vi "load_standards.vi"(10 "Standards Tree ref":refnum<vi>) -> ()   [LabVIEW 2017]
doc: "loads the Standards information from the StabdardsObjects (NOT from the Standards.ini)"
uses:
  global variables.vi
  Classes/Standard/Standard.lvclass
panel:
  out "error out":errorcluster
  in  "error in (no error)":errorcluster
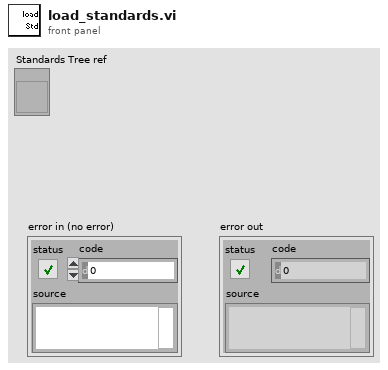
[diagram p1: front panel]
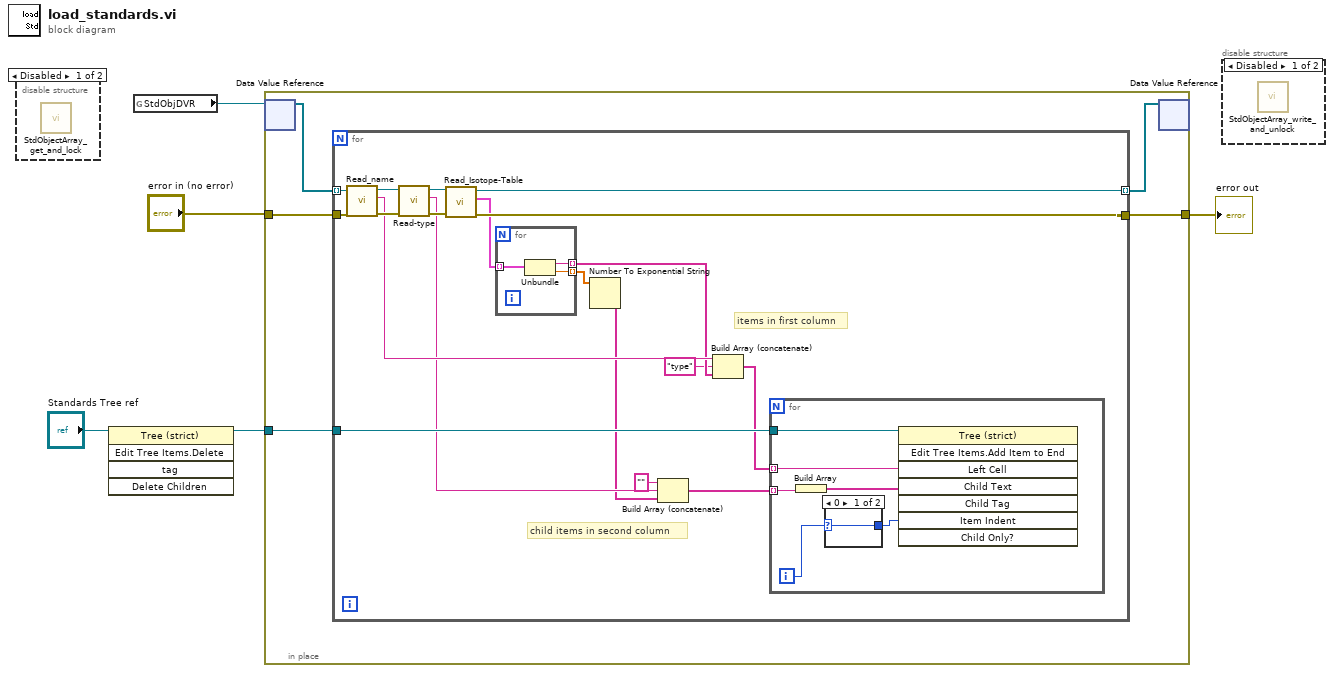
[diagram p0: block diagram]
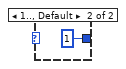
[diagram p4: hidden frame]
diagram:
  n1 = disable-structure shown="Disabled" {
    frame Disabled {
      n2 = call "StdObjectArray_get_and_lock.vi"() -> ()  [unwired: 10 in, 2 out]
    }
    frame Enabled {
    }
  }
  n3 = invoke on="Invoke Node" class="Tree (strict)" method="Edit Tree Items.Delete"(reference="Standards Tree ref") -> (reference out=w4:refnum<vi>)  [unwired: 4 in, 4 out]
  n4 = global read "global variables.vi" "StdObjDVR"() -> (w3:refnum<data-value>)
  n5 = in-place {
    in-place-border: [w10] -> w2
    in-place-border: "error in (no error)" -> [w9]
    in-place-border: w4 -> [w8]
    n6 = in-place-dvr #1(w3) -> (w7:refnum<class "Standard.lvclass">[])  [unwired: 1 out]
    n7 = for {
      tunnel: w7 -> [w29] mode=indexing
      tunnel: [w26] -> w6 mode=indexing
      tunnel: w9 -> [w25]
      tunnel: [w22] -> w10
      tunnel: w8 -> [w21]
      # "child items in second column"
      # "items in first column"
      n8 = call-dynamic "Read_name.vi"("error in (no error)"=w25, "Standard in"=w29) -> ("error out"=w24:errorcluster, "standard name"=w20:string, "Standard out"=w28:refnum<class "Standard.lvclass">)  [unwired: 7 in]
      n9 = call-dynamic "Read-type.vi"("error in (no error)"=w24, "Standard in"=w28) -> ("error out"=w23:errorcluster, "type"=w14:string, "Standard out"=w27:refnum<class "Standard.lvclass">)  [unwired: 7 in]
      n10 = call-dynamic "Read_Isotope-Table.vi"("error in (no error)"=w23, "Standard in"=w27) -> ("error out"=w22:errorcluster, "Isotope Table"=w19:cluster{"isotope":string, "amount cc":dbl}[], "Standard out"=w26:refnum<class "Standard.lvclass">)  [unwired: 7 in]
      n11 = for {
        tunnel: w19 -> [w40] mode=indexing
        tunnel: [w39] -> w18 mode=indexing
        tunnel: [w38] -> w17 mode=indexing
        n12 = Unbundle(w40) -> ("isotope"=w39:string, "amount cc"=w38:dbl)
      }
      n13 = Number To Exponential String(number=w17) -> (E-format string=w13:string[])  [unwired: 3 in]
      n14 = Build Array (concatenate)("" ("element"), w14, w13) -> (w11:string[])
      n15 = Build Array (concatenate)(w20, "type" ("element"), w18) -> (w16:string[])
      n16 = for {
        tunnel: w21 -> [w35]
        tunnel: w16 -> [w34] mode=indexing
        tunnel: w11 -> [w31] mode=indexing
        i -> [w33]
        n17 = Build Array(w31) -> (w30:string[])
        n18 = case shown="0" w33 {
          selector: w33 -> [w36 _]
          tunnel: [w36 1] -> w32
          frame 0 {
          }
          frame 1.., Default {
          }
        }
        n19 = invoke class="Tree (strict)" method="Edit Tree Items.Add Item to End"(reference=w35, "Left Cell"=w34, "Child Text"=w30, "Item Indent"=w32) -> ()  [unwired: 4 in, 8 out]
      }
    }
    n20 = in-place-dvr #1(w6) -> ()  [unwired: 2 out]
  }
  "error out" <- w2
  n21 = disable-structure shown="Disabled" {
    frame Disabled {
      n22 = call "StdObjectArray_write_and_unlock.vi"() -> ()  [unwired: 11 in, 1 out]
    }
    frame Enabled {
    }
  }
